vi "Get Int.vi"(8 "error in (no error)":errorcluster, 11 "IIntByVal in":refnum<class "IIntByVal.lvclass">) -> (0 "error out":errorcluster, 2 "Int":i32, 3 "IIntByVal out":refnum<class "IIntByVal.lvclass">)   [LabVIEW 2009, in "IIntByVal.lvclass"]
uses:
  IIntByVal.lvclass
  Numeric Test Object.lvclass
  Source/IUnknown Class/IUnknown.lvclass
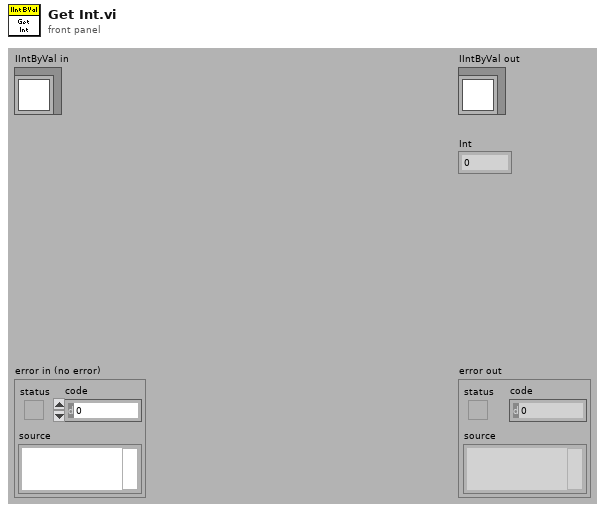
[diagram p1: front panel]
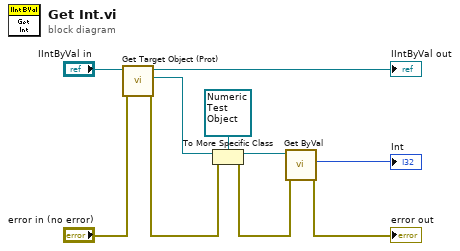
[diagram p0: block diagram]
diagram:
  n1 = call "Get Target Object (Prot).vi"("error in (no error)"="error in (no error)", "IUnknown in"="IIntByVal in") -> ("error out"=w5:errorcluster, "Target Object"=w7:refnum<class "Interfaceable.lvclass">, "IUnknown out"=→"IIntByVal out":refnum<class "IIntByVal.lvclass">)  [unwired: 7 in]
  n2 = To More Specific Class(target class=refnum<class "Numeric Test Object.lvclass"> refnum ("Numeric.lvclass"), reference=w7, error in=w5) -> (specific class reference=w4:refnum<class "Numeric Test Object.lvclass">, error out=w3:errorcluster)
  n3 = call-dynamic "Get ByVal.vi"("error in (no error)"=w3, "Numeric in"=w4) -> ("error out"=→"error out":errorcluster, "Int"=→"Int":i32)  [unwired: 7 in, 1 out]
